vi "Drum Subvi.vi"(0 "Yellow Line":T2={"Global Rectangle"=[342, 292, 349, 377], "Contours"=[{"ID"=enum."External", "Type"=2, "Coordinates"=[342, 376, 348, 292]}]} {"Contours"."Type" items=["No Selection", "Point", "Line", "Rectangle", "Oval", "Polygon", "Freehand Region", "Annulus", "Unused2", "Unused3", "Broken Line", "Freehand Line", "Rotated Rectangle"]}, 1 "Green Line":T2={"Global Rectangle"=[406, 309, 423, 383], "Contours"=[{"ID"=enum."External", "Type"=2, "Coordinates"=[422, 382, 406, 309]}]} {"Contours"."Type" items=["No Selection", "Point", "Line", "Rectangle", "Oval", "Polygon", "Freehand Region", "Annulus", "Unused2", "Unused3", "Broken Line", "Freehand Line", "Rotated Rectangle"]}, 3 "Red Line":T2={"Global Rectangle"=[300, 297, 320, 380], "Contours"=[{"ID"=enum."External", "Type"=2, "Coordinates"=[300, 379, 319, 297]}]} {"Contours"."Type" items=["No Selection", "Point", "Line", "Rectangle", "Oval", "Polygon", "Freehand Region", "Annulus", "Unused2", "Unused3", "Broken Line", "Freehand Line", "Rotated Rectangle"]}, 8 "Image Dst Out":T1, 12 "Blue Line":T2={"Global Rectangle"=[374, 278, 383, 377], "Contours"=[{"ID"=enum."External", "Type"=2, "Coordinates"=[382, 376, 374, 278]}]} {"Contours"."Type" items=["No Selection", "Point", "Line", "Rectangle", "Oval", "Polygon", "Freehand Region", "Annulus", "Unused2", "Unused3", "Broken Line", "Freehand Line", "Rotated Rectangle"]}, 14 "error out":errorcluster) -> (4 "Waveform Red":dbl[](graph), 5 "Boolean":bool, 7 "LED Red":bool, 9 "Waveform Green":dbl[](graph), 13 "Boolean 2":bool, 15 "Boolean 3":bool, 16 "Boolean array":bool[](array[boolean]), 17 "Boolean 4":bool, 20 "Waveform Yellow":dbl[](graph), 22 "Blue Drum":dbl[](graph), 23 "Blue Drum 2":bool, 24 "LED Yellow":bool, 25 "LED Green":bool, 27 "error out 2":errorcluster)   [LabVIEW 2009]
uses:
  <vilib>/vision/Image Controls.llb/IMAQ Image.ctl
  <vilib>/Analysis/3filter.llb/Filter Passband Type.ctl
  <vilib>/Analysis/3filter.llb/Butterworth Filter (DBL).vi
  <vilib>/Analysis/NI_AALBase.lvlib
  <vilib>/vision/NI_Vision_Development_Module.lvlib
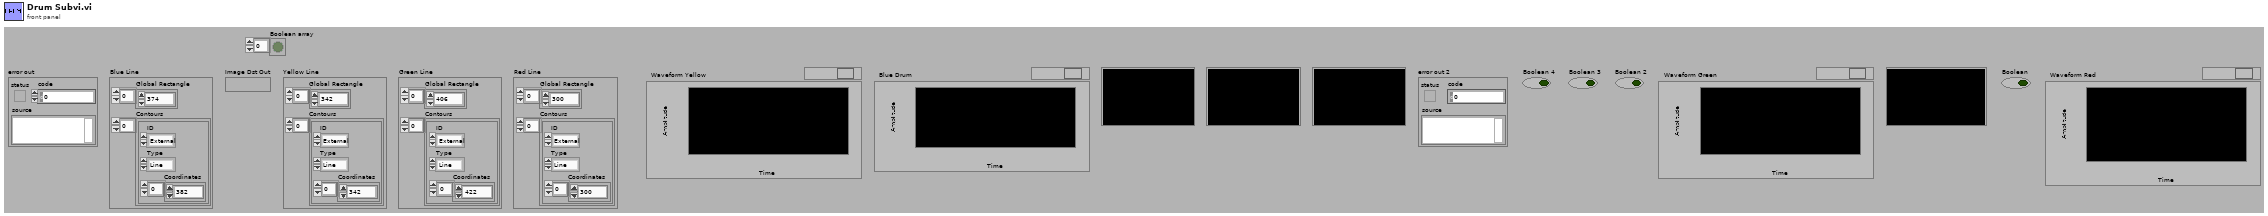
[diagram p1: front panel]
types:
  T1 = typedef "IMAQ Image.ctl" = refnum<image>
  T2 = cluster{"Global Rectangle":i32[], "Contours":cluster{"ID":enum32{"External", "Internal"}, "Type":u32, "Coordinates":i32[]}[]}
  T3 = typedef "NI_AALBase.lvlib/Filter Passband Type.ctl" = enum32{"Lowpass", "Highpass", "Bandpass", "Bandstop"}
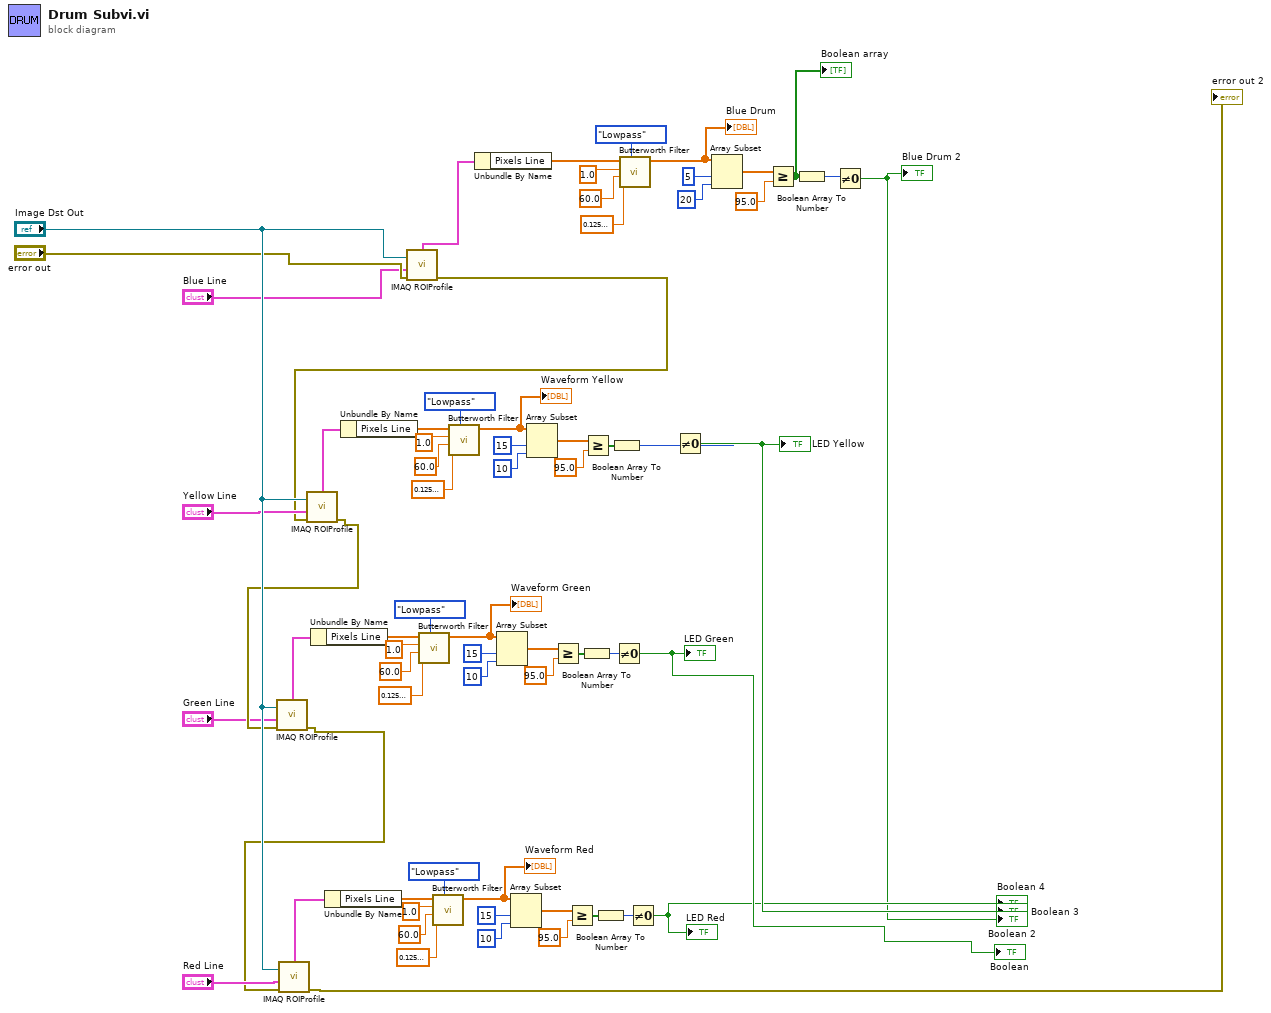
[diagram p0: block diagram]
diagram:
  n1 = call "IMAQ ROIProfile"("error in (no error)"="error out", "ROI Descriptor"="Blue Line", "Image"="Image Dst Out") -> ("error out"=w27:errorcluster, "ROI Graph"=w28:cluster{"x0":sgl, "dx":sgl, "Pixels Line":sgl[]})  [unwired: 4 out]
  n2 = call "IMAQ ROIProfile"("error in (no error)"=w27, "ROI Descriptor"="Yellow Line", "Image"="Image Dst Out") -> ("error out"=w60:errorcluster, "ROI Graph"=w24:cluster{"x0":sgl, "dx":sgl, "Pixels Line":sgl[]})  [unwired: 4 out]
  n3 = call "IMAQ ROIProfile"("error in (no error)"=w60, "ROI Descriptor"="Green Line", "Image"="Image Dst Out") -> ("error out"=w57:errorcluster, "ROI Graph"=w30:cluster{"x0":sgl, "dx":sgl, "Pixels Line":sgl[]})  [unwired: 4 out]
  n4 = call "IMAQ ROIProfile"("error in (no error)"=w57, "ROI Descriptor"="Red Line", "Image"="Image Dst Out") -> ("error out"=→"error out 2":errorcluster, "ROI Graph"=w55:cluster{"x0":sgl, "dx":sgl, "Pixels Line":sgl[]})  [unwired: 4 out]
  n5 = Unbundle By Name(w30) -> ("Pixels Line"=w33:sgl[])
  n6 = Unbundle By Name(w55) -> ("Pixels Line"=w52:sgl[])
  n7 = Unbundle By Name(w24) -> ("Pixels Line"=w21:sgl[])
  n8 = call-poly <vilib>:"Butterworth Filter.vi"("filter type"=Filter_Passband_Type."Lowpass", "low cutoff freq: fl"=0.12500000000000006 ("low  3"), "high cutoff freq: fh"=60.0 ("high 3"), "sampling freq: fs"=1.0 ("sampling 3"), "X"=w33) -> ("Filtered X"=w29:dbl[])  [unwired: 3 in, 1 out]
  "Waveform Green" <- w29
  n9 = call-poly <vilib>:"Butterworth Filter.vi"("filter type"=Filter_Passband_Type."Lowpass", "low cutoff freq: fl"=0.12500000000000006 ("low  4"), "high cutoff freq: fh"=60.0 ("high 4"), "sampling freq: fs"=1.0 ("sampling 4"), "X"=w52) -> ("Filtered X"=w56:dbl[])  [unwired: 3 in, 1 out]
  "Waveform Red" <- w56
  n10 = call-poly <vilib>:"Butterworth Filter.vi"("filter type"=Filter_Passband_Type."Lowpass", "low cutoff freq: fl"=0.12500000000000006 ("low  2"), "high cutoff freq: fh"=60.0 ("high 2"), "sampling freq: fs"=1.0 ("sampling 2"), "X"=w21) -> ("Filtered X"=w25:dbl[])  [unwired: 3 in, 1 out]
  "Waveform Yellow" <- w25
  n11 = Unbundle By Name(w28) -> ("Pixels Line"=w6:sgl[])
  n12 = Array Subset(array=w29, index=15, length=10) -> (w38:dbl[])
  n13 = Array Subset(array=w56, index=15, length=10) -> (w47:dbl[])
  n14 = Array Subset(array=w25, index=15, length=10) -> (w16:dbl[])
  n15 = Greater Or Equal?(x=w38, y=95.0) -> (x >= y?=w36:bool[])
  n16 = Greater Or Equal?(x=w47, y=95.0) -> (x >= y?=w49:bool[])
  n17 = Boolean Array To Number(Boolean array=w36) -> (number=w35:u32)
  n18 = Greater Or Equal?(x=w16, y=95.0) -> (x >= y?=w18:bool[])
  n19 = Boolean Array To Number(Boolean array=w49) -> (number=w50:u32)
  n20 = Boolean Array To Number(Boolean array=w18) -> (number=w19:u32)
  n21 = Not Equal To 0?(x=w35) -> (x != 0?=→"LED Green" →"Boolean":bool)
  n22 = call-poly <vilib>:"Butterworth Filter.vi"("filter type"=Filter_Passband_Type."Lowpass", "low cutoff freq: fl"=0.12500000000000006 ("low"), "high cutoff freq: fh"=60.0 ("high"), "sampling freq: fs"=1.0 ("sampling"), "X"=w6) -> ("Filtered X"=w42:dbl[])  [unwired: 3 in, 1 out]
  "Blue Drum" <- w42
  n23 = Not Equal To 0?(x=w50) -> (x != 0?=→"LED Red" →"Boolean 4":bool)
  n24 = Not Equal To 0?(x=w19) -> (x != 0?=→"LED Yellow" →"Boolean 3":bool)
  n25 = Array Subset(array=w42, index=5, length=20) -> (w12:dbl[])
  n26 = Greater Or Equal?(x=w12, y=95.0) -> (x >= y?=w3:bool[])
  "Boolean array" <- w3
  n27 = Boolean Array To Number(Boolean array=w3) -> (number=w2:u32)
  n28 = Not Equal To 0?(x=w2) -> (x != 0?=→"Blue Drum 2" →"Boolean 2":bool)
